vi "UI Flow Field Flow Rate.vi"(8 "error in":errorcluster) -> (0 "error out":errorcluster)   [LabVIEW 2019, in "Test.lvlib"]
uses:
  Test.lvlib
  Queues/Message Cluster.ctl
  Fluidic Process/SubVI/Fluidic Para.ctl
  LED/SubVI/Image Para.ctl
  MiControl-E/LV Source/ImageSystem/Cradle Zyla_1117/Ctl/seletion.ctl
  <vilib>/Utility/file.llb/Read Delimited Spreadsheet (string).vi
  <vilib>/Utility/error.llb/Error Cluster From Error Code.vi
  <vilib>/ErrorRing/Error Ring.xnode
  Controller/Controller.lvlib
  Queues/Queues.lvlib
  Fluidic Process/Fluidic Process.lvlib
  LED/LED.lvlib
  Motion/Allmotion/Allmotion.lvlib
  Camera/Andor/Andor.lvlib
  Image/Image.lvlib
  Initialize/Initialize.lvlib
panel:
  in  "Locate":bool
  in  "Air Tight":bool
  in  "Stop Process":bool
  out "Remaining Time(s)":dbl
  out "Total Process":string
  out "Current Process":string
  out "Gauge":dbl(knob)=1.2869315802184793e-48 scale=0.0..100.0
  in  "Purge":bool
  in  "Flow Field":bool
  in  "Flow Rate":bool
  in  "Chip Hold Pressure":bool
  in  "Back":bool
  # "/"
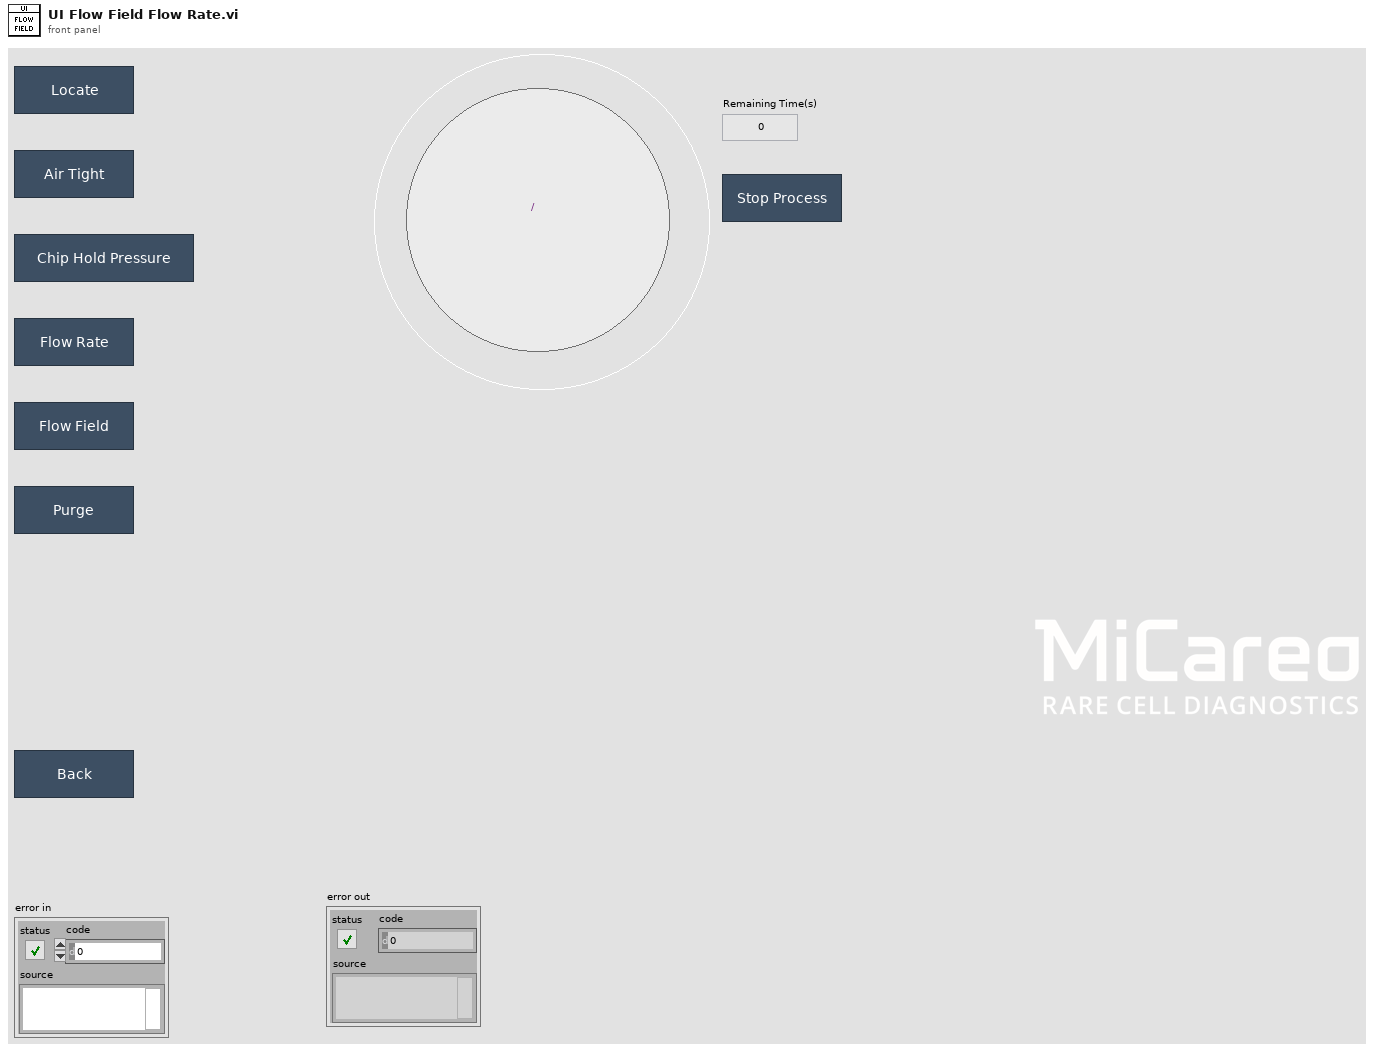
[diagram p1: front panel]
types:
  T1 = cluster{"Tick Count":u32, "Start Time":string, "Round Total":i32, "Round Count":i32, "FOV Offset":i32[], "Current Process":i32, "Take Image Done":bool}
  T2 = cluster{"Flow Field 1":refnum<queue>, "Flow Field 2":refnum<queue>}
  T3 = enum8{"Enabled", "Disabled", "Disabled and Grayed Out"}
  T4 = typedef "Fluidic Process.lvlib/Fluidic Para.ctl" = cluster{"Read Force Sensor":i32, "Read Regulator":i32, "Read Force Sensor?":bool, "Read Regulator?":bool, "Read Syringe Pump":i32, "Read Syringe Pump?":bool}
  T5 = typedef "Fluidic Process.lvlib/SEQ Data.ctl" = cluster{"Fluidic Process Done?":bool, "Current Process":i32, "Remaining Time":dbl, "Total Process":i32, "Air Sealing":bool, "Force Condition":bool}
  T6 = typedef "LED.lvlib/Image Para.ctl" = cluster{"Marker":T7, "Power(Amp)":u8, "set shutter(s)":dbl, "Cube":enum16{"1", "2", "3", "4", "5", "6", "7", "8"}}
  T7 = typedef "seletion.ctl" = enum16{"None", "Red", "Green", "Blue", "UV", "Green Laser", "Blue-Red", "UV-Red", "BF", "UV-IR"}
  T8 = typedef "ROI Descriptor" = cluster{"Global Rectangle":i32[], "Contours":cluster{"ID":enum32{"External", "Internal"}, "Type":u32, "Coordinates":i32[]}[]}
  T9 = cluster{"Image Path":path, "Start Offset":i32, "Template Path":path, "Disable Fine Search":bool, "ROI":T8}
  T10 = typedef "Rendezvous RefNum" = refnum<k1>
  T11 = typedef "Image.lvlib/SEQ Data.ctl" = cluster{"Acquire Done?":bool, "Focus Done?":bool, "Align Done?":bool, "No Position Match?":bool, "Best Wheel Position":string, "Match Done?":bool, "Match Score":dbl, "Focus Score":dbl, "Match Position":cluster{"x":sgl, "y":sgl}, "Flower Position":i32[]}
  T12 = typedef "Allmotion.lvlib/SEQ Data.ctl" = cluster{"Position":i32[], "Arrived?":bool, "VISA name":refnum<visa-resource-name>, "Initialize Done?":bool, "State":string, "VI Refnum":refnum<vi>, "Dichroic Position":string[]}
  T13 = typedef "Initialize.lvlib/SEQ Data.ctl" = cluster{"Folder Path":path}
  T14 = typedef "Andor.lvlib/SEQ Data.ctl" = cluster{"Initialize Sucess?":bool, "Image Ref":T15, "VI Refnum":refnum<vi>}
  T15 = typedef "IMAQ Image.ctl" = refnum<image>
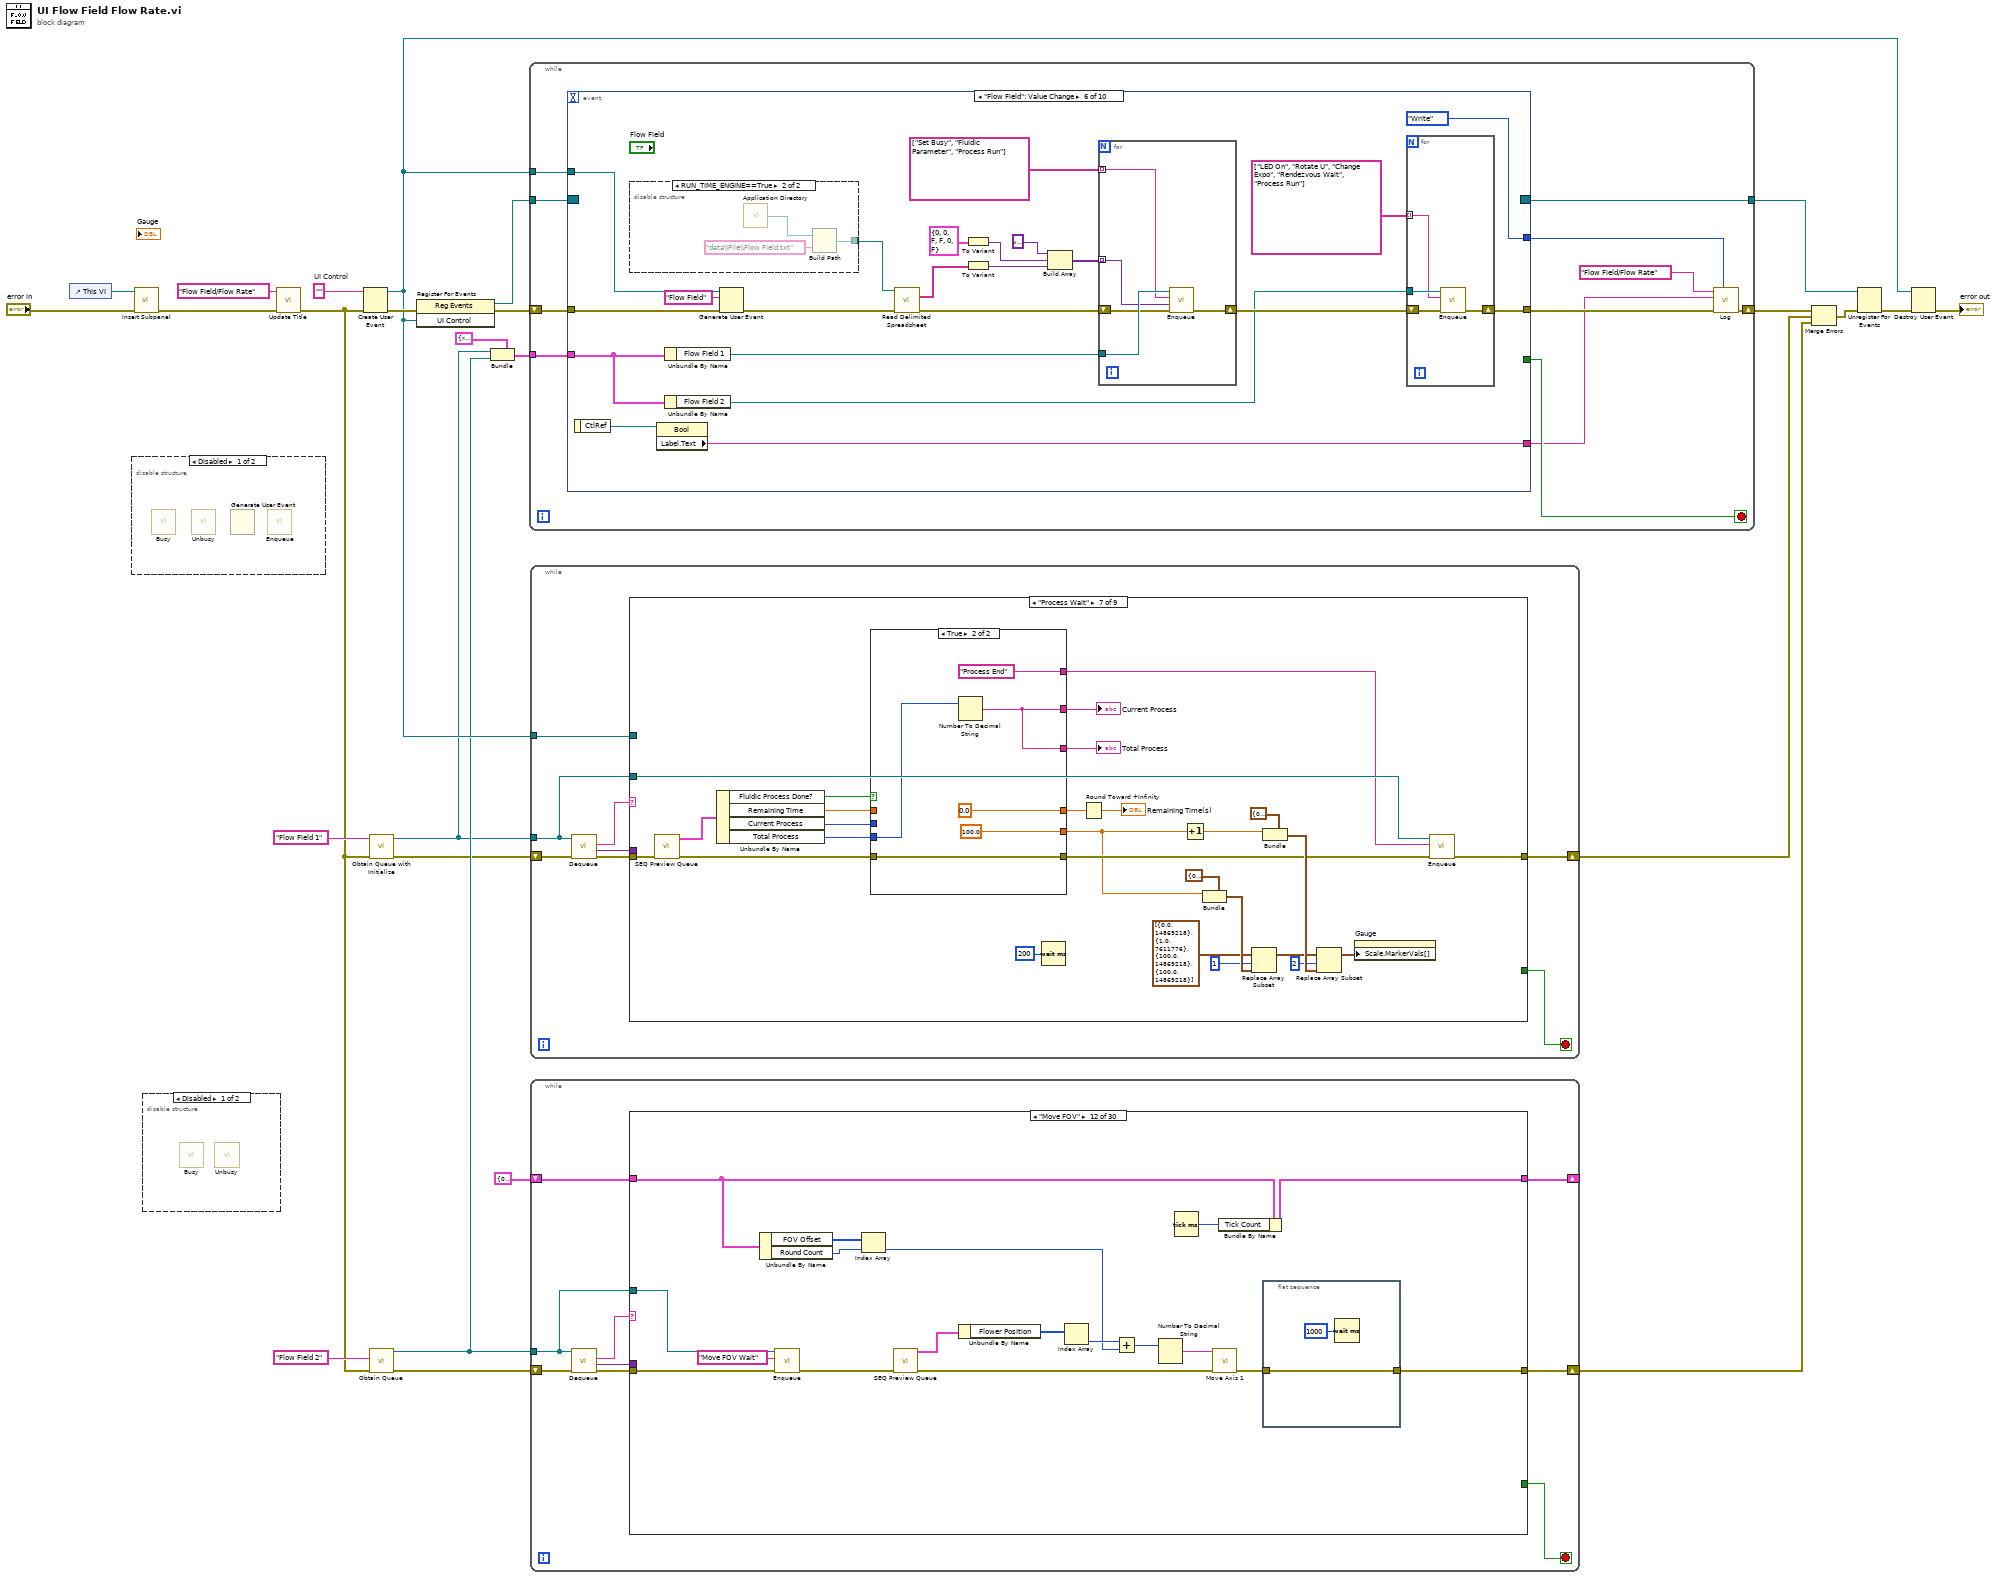
[diagram p0: block diagram]
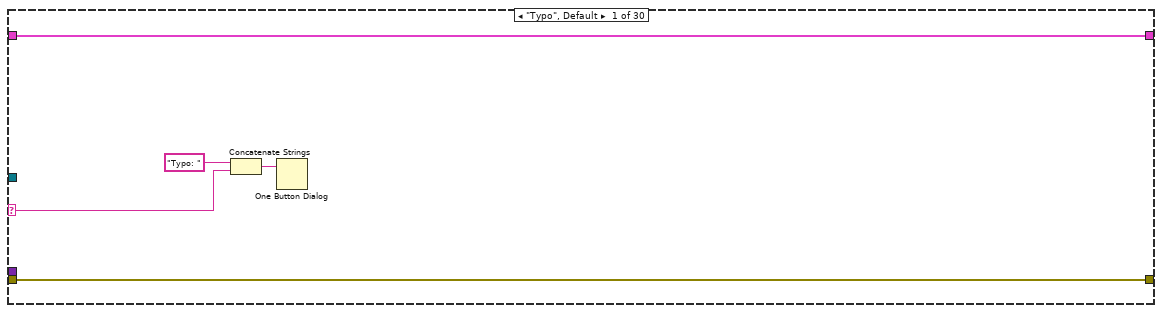
[diagram p3: hidden frame]
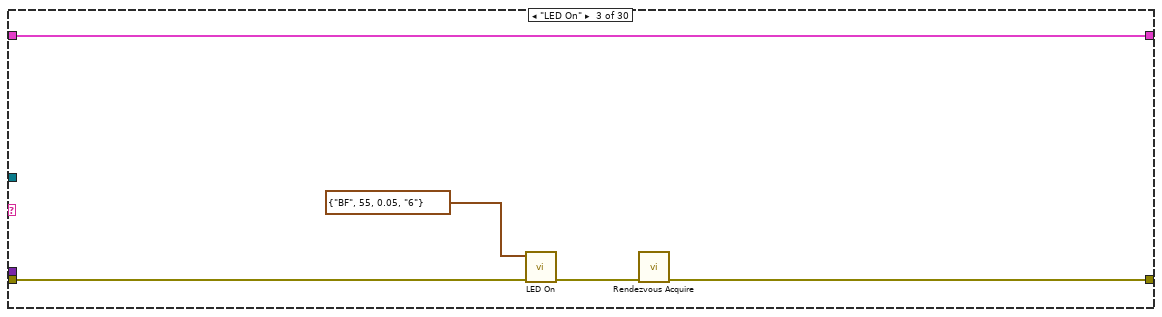
[diagram p5: hidden frame]
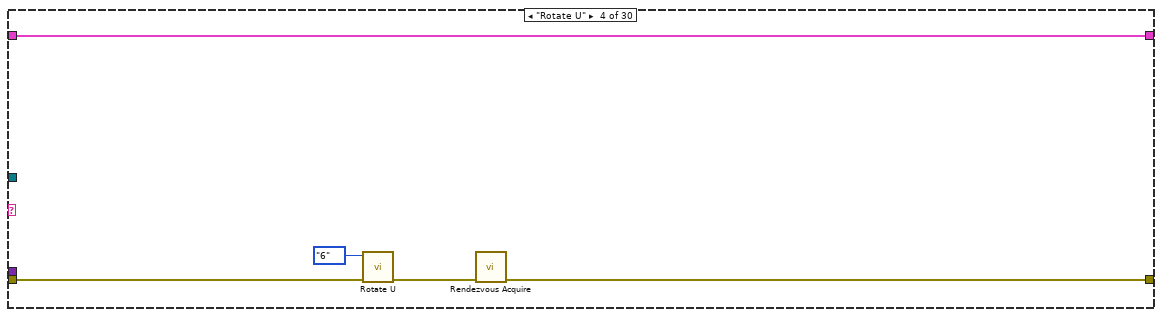
[diagram p6: hidden frame]
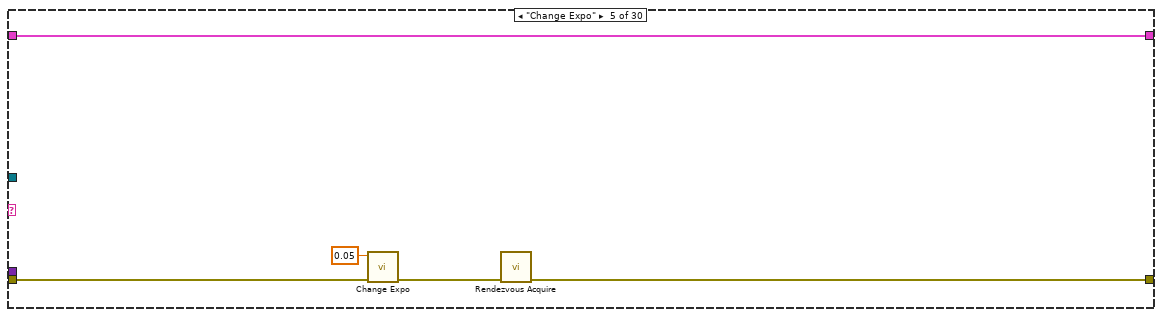
[diagram p7: hidden frame]
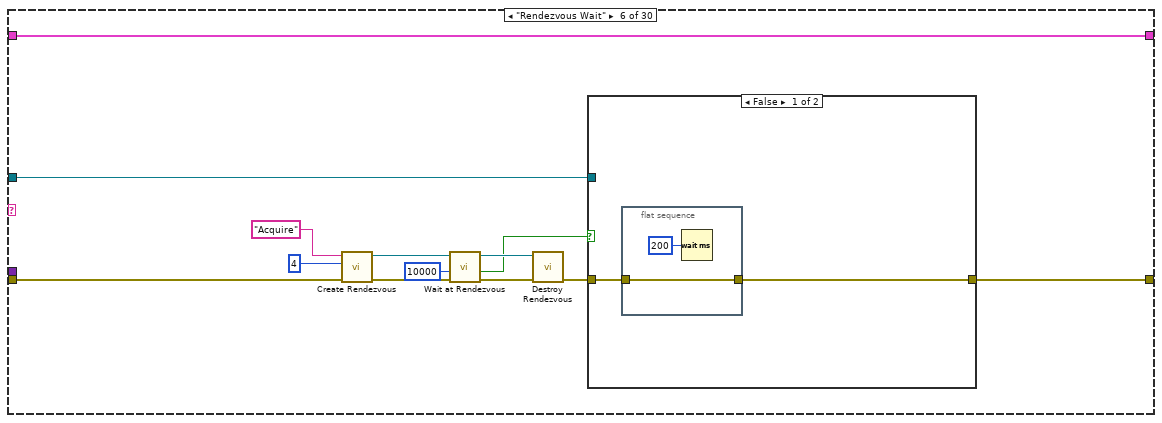
[diagram p8: hidden frame]
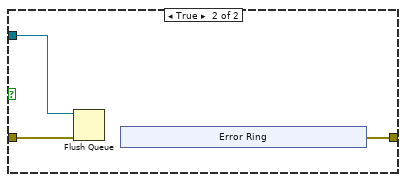
[diagram p9: hidden frame]
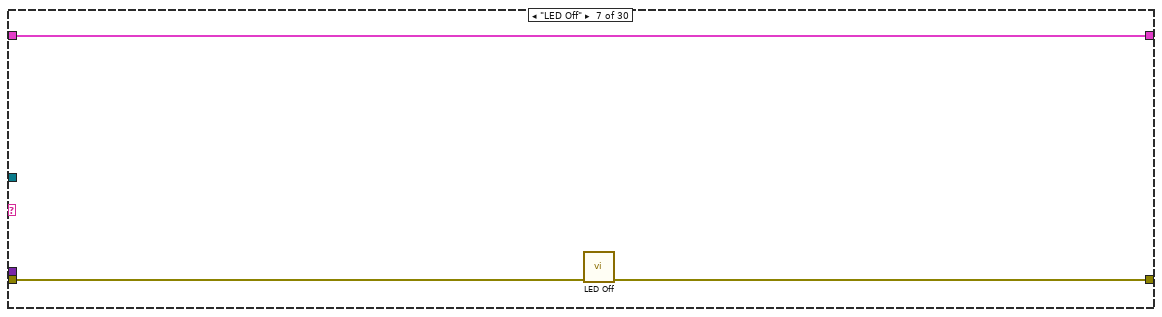
[diagram p10: hidden frame]
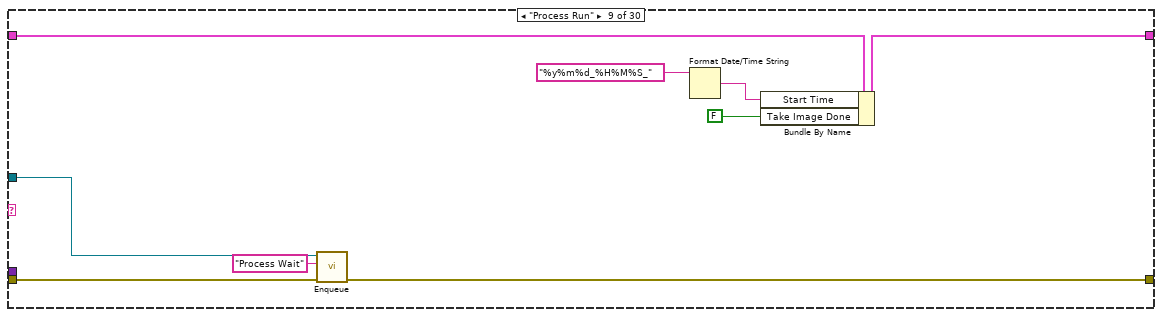
[diagram p12: hidden frame]
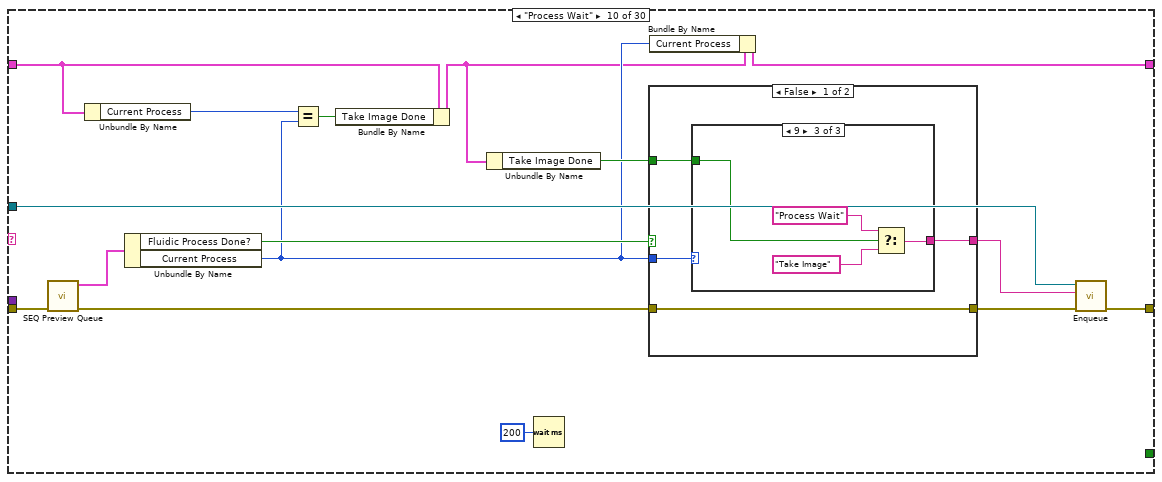
[diagram p13: hidden frame]
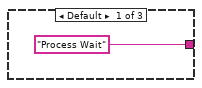
[diagram p14: hidden frame]
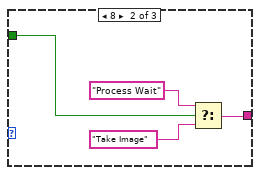
[diagram p15: hidden frame]
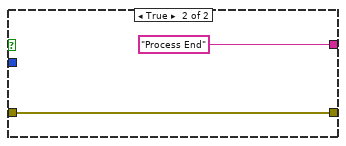
[diagram p16: hidden frame]
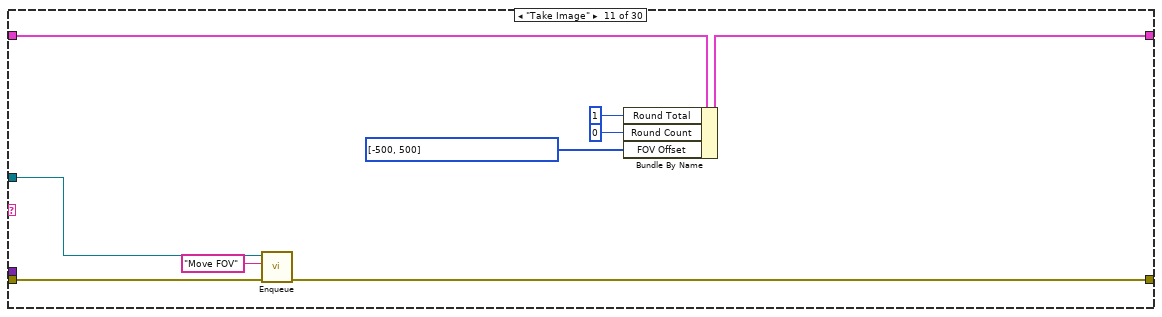
[diagram p17: hidden frame]
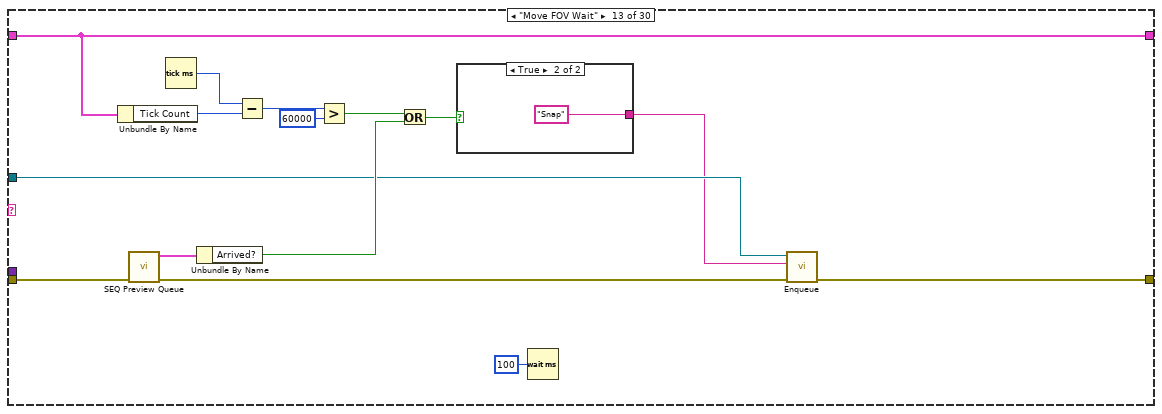
[diagram p18: hidden frame]
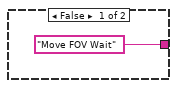
[diagram p19: hidden frame]
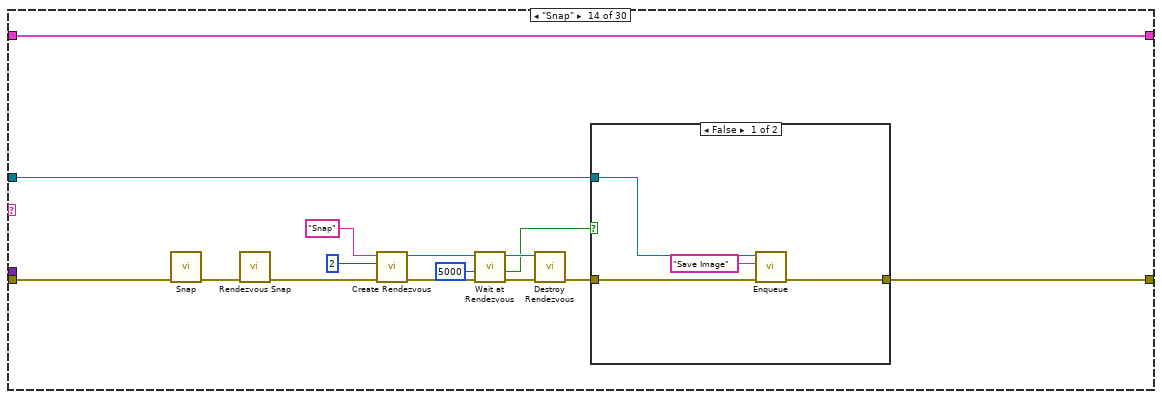
[diagram p20: hidden frame]
diagram:
  w16 = ""  # UI Control
  n1 = control-ref of="This VI"() -> (w15:refnum<vi>)
  n2 = disable-structure shown="Disabled" {
    frame Disabled {
      n3 = call "Busy.vi"() -> ()  [unwired: 11 in, 1 out]
      n4 = call "Unbusy.vi"() -> ()  [unwired: 11 in, 1 out]
      n5 = Generate User Event() -> ()  [unwired: 4 in, 2 out]
      n6 = call "Enqueue.vi"() -> ()  [unwired: 10 in, 2 out]
    }
    frame Enabled {
    }
  }
  n7 = call "Insert Subpanel.vi"("Error In"="error in", "VI Refnum"=w15) -> ("Error Out"=w3:errorcluster)  [unwired: 9 in]
  n8 = disable-structure shown="Disabled" {
    frame Disabled {
      n9 = call "Busy.vi"() -> ()  [unwired: 11 in, 1 out]
      n10 = call "Unbusy.vi"() -> ()  [unwired: 11 in, 1 out]
    }
    frame Enabled {
    }
  }
  n11 = call "Update Title.vi"("Error In"=w3, "Title"="Flow Field/Flow Rate") -> ("Error Out"=w2:errorcluster)  [unwired: 9 in]
  n12 = Create User Event(user event datatype=w16, error in=w2) -> (user event=w12:refnum<user-event>, error out=w25:errorcluster)
  n13 = call "Obtain Queue with Initialize.vi"("Error In"=w2, "Queue Name"="Flow Field 1") -> ("Error Out"=w5:errorcluster, "Queue out"=w4:refnum<queue>)  [unwired: 8 in]
  n14 = call "Obtain Queue.vi"("Error In"=w2, "Queue Name"="Flow Field 2") -> ("Error Out"=w14:errorcluster, "queue out"=w11:refnum<queue>)  [unwired: 8 in]
  n15 = register-events(error in=w25, w12) -> (reference out=w23:refnum<event-registration>, error out=w24:errorcluster)  [unwired: 1 in]
  n16 = Bundle(cluster=T2 {"Flow Field 1"=refnum, "Flow Field 2"=refnum}, "Flow Field 1"=w4, "Flow Field 2"=w11) -> (w9:T2)
  n17 = while {
    tunnel: w23 -> [w35]
    shift-right: [w30] -> w21
    shift-left: w24 -> [w37]
    tunnel: [w34] -> w19
    tunnel: w12 -> [w33]
    tunnel: w9 -> [w32]
    stop <- w36 stop-if-true
    n18 = event shown="[5] \"Flow Field\": Value Change" {
      selector: w35 -> [_ _ _ _ _ _ _ _ _ _]
      dyn-events: [_ _ _ _ _ _ _ _ _ _] -> w34
      timeout: _ -> [_ _ _ _ _ _ _ _ _ _]
      tunnel: w37 -> [w38 w43 w81 w111 w141 w175 w208 w238 w247 w253]
      tunnel: [_ w40 _ _ _ _ _ _ _ TRUE] -> w36
      tunnel: [w38 w41 w89 w119 w149 w170 w216 w237 w246 w254] -> w31
      tunnel: w33 -> [_ _ w79 w109 w139 w173 w206 _ _ _]
      tunnel: w32 -> [_ _ w77 w107 w137 w169 w204 w236 _ w252]
      tunnel: [_ _ w75 w105 w135 w165 w202 w232 w244 w249] -> w28
      tunnel: [_ enum16{"None", "Write"}."None" ("Action") enum16{"None", "Write"}."Write" ("Action") enum16{"None", "Write"}."Write" ("Action") enum16{"None", "Write"}."Write" ("Action") enum16{"None", "Write"}."Write" ("Action") enum16{"None", "Write"}."Write" ("Action") enum16{"None", "Write"}."Write" ("Action") enum16{"None", "Write"}."Write" ("Action") enum16{"None", "Write"}."Write" ("Action")] -> w27
      event Timeout {
        n19 = event-data() -> ()  [unwired: 1 in, 3 out]
      }
      event User Event {
        n20 = event-data() -> ("UI Control"=w42:string)  [unwired: 1 in]
        n21 = case shown="\"Initialize\"" w42 {
          selector: w42 -> [w46 _ _ _ _ _ _ _]
          tunnel: w43 -> [w44 w50 w54 w58 w62 w66 w70 w73]
          tunnel: [w44 w50 w54 w58 w62 w66 w70 w73] -> w41
          tunnel: [TRUE _ _ _ _ _ _ _] -> w40
          frame "Typo", Default {
            n22 = Concatenate Strings("Typo: " ("string"), w46) -> (w47:string)
            n23 = One Button Dialog(message=w47) -> ()  [unwired: 1 in, 1 out]
          }
          frame "Initialize" {
            w49 = T3."Disabled and Grayed Out" ("Disabled")
            n24 = property on="Gauge" class="Knob (strict)"("DisabledEnum"=w49) -> ()  [unwired: 2 in, 2 out]
            n25 = property on="Current Process" class="Str"("DisabledEnum"=w49) -> ()  [unwired: 2 in, 2 out]
            n26 = property on="Total Process" class="Str"("DisabledEnum"=w49) -> ()  [unwired: 2 in, 2 out]
            n27 = property on="Remaining Time(s)" class="DigNum (strict)"("DisabledEnum"=w49) -> ()  [unwired: 2 in, 2 out]
            n28 = property on="Stop Process" class="Bool"("DisabledEnum"=w49) -> ()  [unwired: 2 in, 2 out]
          }
          frame "Chip Hold Pressure" {
            w52 = T3."Enabled" ("Disabled")
            w51 = T3."Disabled and Grayed Out" ("Disabled")
            n29 = property on="Gauge" class="Knob (strict)"("DisabledEnum"=w52) -> ()  [unwired: 2 in, 2 out]
            n30 = property on="Current Process" class="Str"("DisabledEnum"=w52) -> ()  [unwired: 2 in, 2 out]
            n31 = property on="Total Process" class="Str"("DisabledEnum"=w52) -> ()  [unwired: 2 in, 2 out]
            n32 = property on="Remaining Time(s)" class="DigNum (strict)"("DisabledEnum"=w52) -> ()  [unwired: 2 in, 2 out]
            n33 = property on="Stop Process" class="Bool"("DisabledEnum"=w52) -> ()  [unwired: 2 in, 2 out]
            n34 = property on="Chip Hold Pressure" class="Bool"("DisabledEnum"=T3."Enabled" ("Disabled")) -> ()  [unwired: 2 in, 2 out]
            n35 = property on="Flow Rate" class="Bool"("DisabledEnum"=w51) -> ()  [unwired: 2 in, 2 out]
            n36 = property on="Flow Field" class="Bool"("DisabledEnum"=w51) -> ()  [unwired: 2 in, 2 out]
            n37 = property on="Purge" class="Bool"("DisabledEnum"=w51) -> ()  [unwired: 2 in, 2 out]
            n38 = property on="Air Tight" class="Bool"("DisabledEnum"=w51) -> ()  [unwired: 2 in, 2 out]
            n39 = property on="Back" class="Bool"("DisabledEnum"=w51) -> ()  [unwired: 2 in, 2 out]
            n40 = property on="Locate" class="Bool"("DisabledEnum"=w51) -> ()  [unwired: 2 in, 2 out]
          }
          frame "Air Tight" {
            w57 = T3."Enabled" ("Disabled")
            w55 = T3."Disabled and Grayed Out" ("Disabled")
            n41 = property on="Gauge" class="Knob (strict)"("DisabledEnum"=w57) -> ()  [unwired: 2 in, 2 out]
            n42 = property on="Current Process" class="Str"("DisabledEnum"=w57) -> ()  [unwired: 2 in, 2 out]
            n43 = property on="Total Process" class="Str"("DisabledEnum"=w57) -> ()  [unwired: 2 in, 2 out]
            n44 = property on="Remaining Time(s)" class="DigNum (strict)"("DisabledEnum"=w57) -> ()  [unwired: 2 in, 2 out]
            n45 = property on="Stop Process" class="Bool"("DisabledEnum"=w57) -> ()  [unwired: 2 in, 2 out]
            n46 = property on="Chip Hold Pressure" class="Bool"("DisabledEnum"=w55) -> ()  [unwired: 2 in, 2 out]
            n47 = property on="Flow Rate" class="Bool"("DisabledEnum"=w55) -> ()  [unwired: 2 in, 2 out]
            n48 = property on="Flow Field" class="Bool"("DisabledEnum"=w55) -> ()  [unwired: 2 in, 2 out]
            n49 = property on="Purge" class="Bool"("DisabledEnum"=w55) -> ()  [unwired: 2 in, 2 out]
            n50 = property on="Air Tight" class="Bool"("DisabledEnum"=T3."Enabled" ("Disabled")) -> ()  [unwired: 2 in, 2 out]
            n51 = property on="Back" class="Bool"("DisabledEnum"=w55) -> ()  [unwired: 2 in, 2 out]
            n52 = property on="Locate" class="Bool"("DisabledEnum"=w55) -> ()  [unwired: 2 in, 2 out]
          }
          frame "Flow Rate" {
            w60 = T3."Enabled" ("Disabled")
            w59 = T3."Disabled and Grayed Out" ("Disabled")
            n53 = property on="Gauge" class="Knob (strict)"("DisabledEnum"=w60) -> ()  [unwired: 2 in, 2 out]
            n54 = property on="Current Process" class="Str"("DisabledEnum"=w60) -> ()  [unwired: 2 in, 2 out]
            n55 = property on="Total Process" class="Str"("DisabledEnum"=w60) -> ()  [unwired: 2 in, 2 out]
            n56 = property on="Remaining Time(s)" class="DigNum (strict)"("DisabledEnum"=w60) -> ()  [unwired: 2 in, 2 out]
            n57 = property on="Stop Process" class="Bool"("DisabledEnum"=w60) -> ()  [unwired: 2 in, 2 out]
            n58 = property on="Chip Hold Pressure" class="Bool"("DisabledEnum"=w59) -> ()  [unwired: 2 in, 2 out]
            n59 = property on="Flow Rate" class="Bool"("DisabledEnum"=T3."Enabled" ("Disabled")) -> ()  [unwired: 2 in, 2 out]
            n60 = property on="Flow Field" class="Bool"("DisabledEnum"=w59) -> ()  [unwired: 2 in, 2 out]
            n61 = property on="Purge" class="Bool"("DisabledEnum"=w59) -> ()  [unwired: 2 in, 2 out]
            n62 = property on="Air Tight" class="Bool"("DisabledEnum"=w59) -> ()  [unwired: 2 in, 2 out]
            n63 = property on="Back" class="Bool"("DisabledEnum"=w59) -> ()  [unwired: 2 in, 2 out]
            n64 = property on="Locate" class="Bool"("DisabledEnum"=w59) -> ()  [unwired: 2 in, 2 out]
          }
          frame "Flow Field" {
            w64 = T3."Enabled" ("Disabled")
            w63 = T3."Disabled and Grayed Out" ("Disabled")
            n65 = property on="Gauge" class="Knob (strict)"("DisabledEnum"=w64) -> ()  [unwired: 2 in, 2 out]
            n66 = property on="Current Process" class="Str"("DisabledEnum"=w64) -> ()  [unwired: 2 in, 2 out]
            n67 = property on="Total Process" class="Str"("DisabledEnum"=w64) -> ()  [unwired: 2 in, 2 out]
            n68 = property on="Remaining Time(s)" class="DigNum (strict)"("DisabledEnum"=w64) -> ()  [unwired: 2 in, 2 out]
            n69 = property on="Stop Process" class="Bool"("DisabledEnum"=w64) -> ()  [unwired: 2 in, 2 out]
            n70 = property on="Chip Hold Pressure" class="Bool"("DisabledEnum"=w63) -> ()  [unwired: 2 in, 2 out]
            n71 = property on="Flow Rate" class="Bool"("DisabledEnum"=w63) -> ()  [unwired: 2 in, 2 out]
            n72 = property on="Flow Field" class="Bool"("DisabledEnum"=T3."Enabled" ("Disabled")) -> ()  [unwired: 2 in, 2 out]
            n73 = property on="Purge" class="Bool"("DisabledEnum"=w63) -> ()  [unwired: 2 in, 2 out]
            n74 = property on="Air Tight" class="Bool"("DisabledEnum"=w63) -> ()  [unwired: 2 in, 2 out]
            n75 = property on="Back" class="Bool"("DisabledEnum"=w63) -> ()  [unwired: 2 in, 2 out]
            n76 = property on="Locate" class="Bool"("DisabledEnum"=w63) -> ()  [unwired: 2 in, 2 out]
          }
          frame "Purge" {
            w68 = T3."Enabled" ("Disabled")
            w67 = T3."Disabled and Grayed Out" ("Disabled")
            n77 = property on="Gauge" class="Knob (strict)"("DisabledEnum"=w68) -> ()  [unwired: 2 in, 2 out]
            n78 = property on="Current Process" class="Str"("DisabledEnum"=w68) -> ()  [unwired: 2 in, 2 out]
            n79 = property on="Total Process" class="Str"("DisabledEnum"=w68) -> ()  [unwired: 2 in, 2 out]
            n80 = property on="Remaining Time(s)" class="DigNum (strict)"("DisabledEnum"=w68) -> ()  [unwired: 2 in, 2 out]
            n81 = property on="Stop Process" class="Bool"("DisabledEnum"=w68) -> ()  [unwired: 2 in, 2 out]
            n82 = property on="Chip Hold Pressure" class="Bool"("DisabledEnum"=w67) -> ()  [unwired: 2 in, 2 out]
            n83 = property on="Flow Rate" class="Bool"("DisabledEnum"=w67) -> ()  [unwired: 2 in, 2 out]
            n84 = property on="Flow Field" class="Bool"("DisabledEnum"=w67) -> ()  [unwired: 2 in, 2 out]
            n85 = property on="Purge" class="Bool"("DisabledEnum"=T3."Enabled" ("Disabled")) -> ()  [unwired: 2 in, 2 out]
            n86 = property on="Air Tight" class="Bool"("DisabledEnum"=w67) -> ()  [unwired: 2 in, 2 out]
            n87 = property on="Back" class="Bool"("DisabledEnum"=w67) -> ()  [unwired: 2 in, 2 out]
            n88 = property on="Locate" class="Bool"("DisabledEnum"=w67) -> ()  [unwired: 2 in, 2 out]
          }
          frame "Process End" {
            w72 = T3."Disabled and Grayed Out" ("Disabled")
            w71 = T3."Enabled" ("Disabled")
            n89 = property on="Gauge" class="Knob (strict)"("DisabledEnum"=w72) -> ()  [unwired: 2 in, 2 out]
            n90 = property on="Current Process" class="Str"("DisabledEnum"=w72) -> ()  [unwired: 2 in, 2 out]
            n91 = property on="Total Process" class="Str"("DisabledEnum"=w72) -> ()  [unwired: 2 in, 2 out]
            n92 = property on="Remaining Time(s)" class="DigNum (strict)"("DisabledEnum"=w72) -> ()  [unwired: 2 in, 2 out]
            n93 = property on="Stop Process" class="Bool"("DisabledEnum"=w72) -> ()  [unwired: 2 in, 2 out]
            n94 = property on="Chip Hold Pressure" class="Bool"("DisabledEnum"=w71) -> ()  [unwired: 2 in, 2 out]
            n95 = property on="Flow Rate" class="Bool"("DisabledEnum"=w71) -> ()  [unwired: 2 in, 2 out]
            n96 = property on="Flow Field" class="Bool"("DisabledEnum"=w71) -> ()  [unwired: 2 in, 2 out]
            n97 = property on="Purge" class="Bool"("DisabledEnum"=w71) -> ()  [unwired: 2 in, 2 out]
            n98 = property on="Air Tight" class="Bool"("DisabledEnum"=w71) -> ()  [unwired: 2 in, 2 out]
            n99 = property on="Back" class="Bool"("DisabledEnum"=w71) -> ()  [unwired: 2 in, 2 out]
            n100 = property on="Locate" class="Bool"("DisabledEnum"=w71) -> ()  [unwired: 2 in, 2 out]
          }
        }
      }
      event "Chip Hold Pressure": Value Change {
        n101 = event-data() -> ("CtlRef"=w76:refnum<vi>)  [unwired: 1 in]
        n102 = property class="Bool"(reference=w76) -> ("Label.Text"=w75:string)  [unwired: 1 in, 2 out]
        n103 = Unbundle By Name(w77) -> ("Flow Field 1"=w78:refnum<queue>)
        n104 = disable-structure shown="RUN_TIME_ENGINE==True" {
          disable-tunnel: [w93 w96] -> w91
          frame condition #0 (active) {
            n105 = call <vilib>:"Application Directory.vi"() -> ("Application Directory"=w95:path)
            n106 = Build Path(base path=w95, name or relative path="Fluidic Process\\File\\Chip Hold Pressure.txt") -> (appended path=w93:path)
          }
          frame condition #1 {
            n107 = call <vilib>:"Application Directory.vi"() -> ("Application Directory"=w98:path)
            n108 = Build Path(base path=w98, name or relative path="data\\File\\Chip Hold Pressure.txt") -> (appended path=w96:path)
          }
        }
        n109 = Generate User Event(user event=w79, event data cluster="Chip Hold Pressure" ("event data"), error in=w81) -> (error out=w80:errorcluster)  [unwired: 1 in, 1 out]
        n110 = call-poly <vilib>:"Read Delimited Spreadsheet.vi"("file path (dialog if empty)"=w91, "error in (no error)"=w80) -> ("all rows"=w90:string[][], "error out"=w92:errorcluster)  [unwired: 8 in, 4 out]
        n111 = To Variant(anything=T4 {"Read Force Sensor"=0, "Read Regulator"=0, "Read Force Sensor?"=FALSE, "Read Regulator?"=FALSE, "Read Syringe Pump"=0, "Read Syringe Pump?"=FALSE} ("Cluster")) -> (Variant=w85:variant)
        n112 = To Variant(anything=w90) -> (Variant=w87:variant)
        n113 = Build Array(variant, w85, w87) -> (w84:variant[])
        n114 = for {
          tunnel: w78 -> [w103]
          shift-right: [w101] -> w89
          shift-left: w92 -> [w102]
          tunnel: string[] ["Set Busy", "Fluidic Parameter", "Process Run"] -> [w100] mode=indexing
          tunnel: w84 -> [w99] mode=indexing
          n115 = call "Enqueue.vi"("Error In"=w102, "Data"=w99, "State"=w100, "Queue in"=w103) -> ("Error Out"=w101:errorcluster)  [unwired: 6 in, 1 out]
        }
      }
      event "Air Tight": Value Change {
        n116 = event-data() -> ("CtlRef"=w106:refnum<vi>)  [unwired: 1 in]
        n117 = Unbundle By Name(w107) -> ("Flow Field 1"=w108:refnum<queue>)
        n118 = property class="Bool"(reference=w106) -> ("Label.Text"=w105:string)  [unwired: 1 in, 2 out]
        n119 = Generate User Event(user event=w109, event data cluster="Air Tight" ("event data"), error in=w111) -> (error out=w110:errorcluster)  [unwired: 1 in, 1 out]
        n120 = disable-structure shown="RUN_TIME_ENGINE==False, Default" {
          disable-tunnel: [w123 w126] -> w121
          frame condition #0 (active) {
            n121 = call <vilib>:"Application Directory.vi"() -> ("Application Directory"=w125:path)
            n122 = Build Path(base path=w125, name or relative path="Fluidic Process\\File\\Air Tight.txt") -> (appended path=w123:path)
          }
          frame condition #1 {
            n123 = call <vilib>:"Application Directory.vi"() -> ("Application Directory"=w128:path)
            n124 = Build Path(base path=w128, name or relative path="data\\File\\Air Tight.txt") -> (appended path=w126:path)
          }
        }
        n125 = call-poly <vilib>:"Read Delimited Spreadsheet.vi"("file path (dialog if empty)"=w121, "error in (no error)"=w110) -> ("all rows"=w120:string[][], "error out"=w122:errorcluster)  [unwired: 8 in, 4 out]
        n126 = To Variant(anything=T4 {"Read Force Sensor"=0, "Read Regulator"=2, "Read Force Sensor?"=FALSE, "Read Regulator?"=TRUE, "Read Syringe Pump"=0, "Read Syringe Pump?"=FALSE} ("Cluster")) -> (Variant=w115:variant)
        n127 = To Variant(anything=w120) -> (Variant=w117:variant)
        n128 = Build Array(variant, w115, w117) -> (w114:variant[])
        n129 = for {
          tunnel: w108 -> [w133]
          shift-right: [w131] -> w119
          shift-left: w122 -> [w132]
          tunnel: string[] ["Set Busy", "Fluidic Parameter", "Process Run"] -> [w130] mode=indexing
          tunnel: w114 -> [w129] mode=indexing
          n130 = call "Enqueue.vi"("Error In"=w132, "Data"=w129, "State"=w130, "Queue in"=w133) -> ("Error Out"=w131:errorcluster)  [unwired: 6 in, 1 out]
        }
      }
      event "Flow Rate": Value Change {
        n131 = event-data() -> ("CtlRef"=w136:refnum<vi>)  [unwired: 1 in]
        n132 = Unbundle By Name(w137) -> ("Flow Field 1"=w138:refnum<queue>)
        n133 = property class="Bool"(reference=w136) -> ("Label.Text"=w135:string)  [unwired: 1 in, 2 out]
        n134 = Generate User Event(user event=w139, event data cluster="Flow Rate" ("event data"), error in=w141) -> (error out=w140:errorcluster)  [unwired: 1 in, 1 out]
        n135 = disable-structure shown="RUN_TIME_ENGINE==True" {
          disable-tunnel: [w153 w156] -> w151
          frame condition #0 (active) {
            n136 = call <vilib>:"Application Directory.vi"() -> ("Application Directory"=w155:path)
            n137 = Build Path(base path=w155, name or relative path="Fluidic Process\\File\\Flow Rate.txt") -> (appended path=w153:path)
          }
          frame condition #1 {
            n138 = call <vilib>:"Application Directory.vi"() -> ("Application Directory"=w158:path)
            n139 = Build Path(base path=w158, name or relative path="data\\File\\Flow Rate.txt") -> (appended path=w156:path)
          }
        }
        n140 = call-poly <vilib>:"Read Delimited Spreadsheet.vi"("file path (dialog if empty)"=w151, "error in (no error)"=w140) -> ("all rows"=w150:string[][], "error out"=w152:errorcluster)  [unwired: 8 in, 4 out]
        n141 = To Variant(anything=T4 {"Read Force Sensor"=0, "Read Regulator"=0, "Read Force Sensor?"=FALSE, "Read Regulator?"=FALSE, "Read Syringe Pump"=0, "Read Syringe Pump?"=FALSE} ("Cluster")) -> (Variant=w145:variant)
        n142 = To Variant(anything=w150) -> (Variant=w147:variant)
        n143 = Build Array(variant, w145, w147) -> (w144:variant[])
        n144 = for {
          tunnel: w138 -> [w163]
          shift-right: [w161] -> w149
          shift-left: w152 -> [w162]
          tunnel: string[] ["Set Busy", "Fluidic Parameter", "Process Run"] -> [w160] mode=indexing
          tunnel: w144 -> [w159] mode=indexing
          n145 = call "Enqueue.vi"("Error In"=w162, "Data"=w159, "State"=w160, "Queue in"=w163) -> ("Error Out"=w161:errorcluster)  [unwired: 6 in, 1 out]
        }
      }
      event "Flow Field": Value Change {
        n146 = event-data() -> ("CtlRef"=w166:refnum<vi>)  [unwired: 1 in]
        n147 = disable-structure shown="RUN_TIME_ENGINE==True" {
          disable-tunnel: [w190 w193] -> w184
          frame condition #0 (active) {
            n148 = call <vilib>:"Application Directory.vi"() -> ("Application Directory"=w192:path)
            n149 = Build Path(base path=w192, name or relative path="Fluidic Process\\File\\Flow Field.txt") -> (appended path=w190:path)
          }
          frame condition #1 {
            n150 = call <vilib>:"Application Directory.vi"() -> ("Application Directory"=w195:path)
            n151 = Build Path(base path=w195, name or relative path="data\\File\\Flow Field.txt") -> (appended path=w193:path)
          }
        }
        n152 = property class="Bool"(reference=w166) -> ("Label.Text"=w165:string)  [unwired: 1 in, 2 out]
        n153 = Unbundle By Name(w169) -> ("Flow Field 1"=w172:refnum<queue>)
        n154 = Unbundle By Name(w169) -> ("Flow Field 2"=w168:refnum<queue>)
        n155 = Generate User Event(user event=w173, event data cluster="Flow Field" ("event data"), error in=w175) -> (error out=w174:errorcluster)  [unwired: 1 in, 1 out]
        n156 = call-poly <vilib>:"Read Delimited Spreadsheet.vi"("file path (dialog if empty)"=w184, "error in (no error)"=w174) -> ("all rows"=w183:string[][], "error out"=w185:errorcluster)  [unwired: 8 in, 4 out]
        n157 = To Variant(anything=T4 {"Read Force Sensor"=0, "Read Regulator"=0, "Read Force Sensor?"=FALSE, "Read Regulator?"=FALSE, "Read Syringe Pump"=0, "Read Syringe Pump?"=FALSE} ("Cluster")) -> (Variant=w179:variant)
        n158 = To Variant(anything=w183) -> (Variant=w181:variant)
        n159 = Build Array(variant, w179, w181) -> (w178:variant[])
        n160 = for {
          tunnel: w172 -> [w200]
          shift-right: [w198] -> w171
          shift-left: w185 -> [w199]
          tunnel: string[] ["Set Busy", "Fluidic Parameter", "Process Run"] -> [w197] mode=indexing
          tunnel: w178 -> [w196] mode=indexing
          n161 = call "Enqueue.vi"("Error In"=w199, "Data"=w196, "State"=w197, "Queue in"=w200) -> ("Error Out"=w198:errorcluster)  [unwired: 6 in, 1 out]
        }
        n162 = for {
          tunnel: w168 -> [w187]
          shift-right: [w188] -> w170
          shift-left: w171 -> [w189]
          tunnel: string[] ["LED On", "Rotate U", "Change Expo", "Rendezvous Wait", "Process Run"] -> [w186] mode=indexing
          n163 = call "Enqueue.vi"("Error In"=w189, "State"=w186, "Queue in"=w187) -> ("Error Out"=w188:errorcluster)  [unwired: 7 in, 1 out]
        }
      }
      event "Purge": Value Change {
        n164 = event-data() -> ("CtlRef"=w203:refnum<vi>)  [unwired: 1 in]
        n165 = property class="Bool"(reference=w203) -> ("Label.Text"=w202:string)  [unwired: 1 in, 2 out]
        n166 = Unbundle By Name(w204) -> ("Flow Field 1"=w205:refnum<queue>)
        n167 = Generate User Event(user event=w206, event data cluster="Purge" ("event data"), error in=w208) -> (error out=w207:errorcluster)  [unwired: 1 in, 1 out]
        n168 = disable-structure shown="RUN_TIME_ENGINE==False, Default" {
          disable-tunnel: [w220 w223] -> w218
          frame condition #0 (active) {
            n169 = call <vilib>:"Application Directory.vi"() -> ("Application Directory"=w222:path)
            n170 = Build Path(base path=w222, name or relative path="Fluidic Process\\File\\Purge.txt") -> (appended path=w220:path)
          }
          frame condition #1 {
            n171 = call <vilib>:"Application Directory.vi"() -> ("Application Directory"=w225:path)
            n172 = Build Path(base path=w225, name or relative path="data\\File\\Purge.txt") -> (appended path=w223:path)
          }
        }
        n173 = call-poly <vilib>:"Read Delimited Spreadsheet.vi"("file path (dialog if empty)"=w218, "error in (no error)"=w207) -> ("all rows"=w217:string[][], "error out"=w219:errorcluster)  [unwired: 8 in, 4 out]
        n174 = To Variant(anything=T4 {"Read Force Sensor"=0, "Read Regulator"=0, "Read Force Sensor?"=FALSE, "Read Regulator?"=FALSE, "Read Syringe Pump"=3, "Read Syringe Pump?"=TRUE} ("Cluster")) -> (Variant=w212:variant)
        n175 = To Variant(anything=w217) -> (Variant=w214:variant)
        n176 = Build Array(variant, w212, w214) -> (w211:variant[])
        n177 = for {
          tunnel: w205 -> [w230]
          shift-right: [w228] -> w216
          shift-left: w219 -> [w229]
          tunnel: string[] ["Set Busy", "Fluidic Parameter", "Process Run"] -> [w227] mode=indexing
          tunnel: w211 -> [w226] mode=indexing
          n178 = call "Enqueue.vi"("Error In"=w229, "Data"=w226, "State"=w227, "Queue in"=w230) -> ("Error Out"=w228:errorcluster)  [unwired: 6 in, 1 out]
        }
      }
      event "Locate": Value Change {
        n179 = event-data() -> ("CtlRef"=w233:refnum<vi>)  [unwired: 1 in]
        n180 = property class="Bool"(reference=w233) -> ("Label.Text"=w232:string)  [unwired: 1 in, 2 out]
        n181 = Unbundle By Name(w236) -> ("Flow Field 2"=w235:refnum<queue>)
        n182 = for {
          tunnel: w235 -> [w240]
          shift-right: [w241] -> w237
          shift-left: w238 -> [w242]
          tunnel: string[] ["LED On", "Rotate U", "Change Expo", "Rendezvous Wait", "Go Reference"] -> [w239] mode=indexing
          n183 = call "Enqueue.vi"("Error In"=w242, "State"=w239, "Queue in"=w240) -> ("Error Out"=w241:errorcluster)  [unwired: 7 in, 1 out]
        }
      }
      event "Stop Process": Value Change {
        n184 = event-data() -> ("CtlRef"=w245:refnum<vi>)  [unwired: 1 in]
        n185 = property class="Bool"(reference=w245) -> ("Label.Text"=w244:string)  [unwired: 1 in, 2 out]
        n186 = call "Stop Process.vi"("Error In"=w247) -> ("Error Out"=w246:errorcluster)  [unwired: 10 in]
      }
      event "Back": Value Change {
        n187 = event-data() -> ("CtlRef"=w250:refnum<vi>)  [unwired: 1 in]
        n188 = property class="Bool"(reference=w250) -> ("Label.Text"=w249:string)  [unwired: 1 in, 2 out]
        n189 = Cluster To Array(cluster=w252) -> (array=w251:refnum<queue>[])
        n190 = for {
          shift-right: [w259] -> w254
          shift-left: w253 -> [w258]
          tunnel: w251 -> [w257] mode=indexing
          n191 = call "Enqueue.vi"("Error In"=w258, "State"="Close", "Queue in"=w257) -> ("Error Out"=w259:errorcluster)  [unwired: 7 in, 1 out]
        }
      }
    }
    n192 = call "Log.vi"("Action"=w27, "error in"=w31, "State"=w28, "Page Name"="Flow Field/Flow Rate") -> ("error out"=w30:errorcluster)  [unwired: 7 in]
  }
  n193 = while {
    tunnel: w4 -> [w264]
    shift-right: [w262] -> w20
    shift-left: w5 -> [w267]
    tunnel: w12 -> [w261]
    stop <- w260 stop-if-true
    n194 = call "Dequeue.vi"("Error In"=w267, "Queue in"=w264) -> ("Error Out"=w263:errorcluster, "Data"=w265:variant, "State"=w266:string)  [unwired: 6 in, 1 out]
    n195 = case shown="\"Process Wait\"" w266 {
      selector: w266 -> [w269 _ _ _ _ _ _ _ _]
      tunnel: w265 -> [_ _ _ w282 w292 _ _ _ _]
      tunnel: w264 -> [_ _ _ _ w287 w299 w306 _ w349]
      tunnel: w263 -> [w268 w275 w277 w283 w293 w300 w327 w347 w351]
      tunnel: [_ _ _ _ _ _ _ _ TRUE] -> w260
      tunnel: [w268 w274 w276 w278 w284 w296 w311 w346 w350] -> w262
      tunnel: w261 -> [_ w273 _ _ _ _ _ w345 _]
      frame "Typo", Default {
        n196 = Concatenate Strings("Typo: " ("string"), w269) -> (w271:string)
        n197 = One Button Dialog(message=w271) -> ()  [unwired: 1 in, 1 out]
      }
      frame "Initialize" {
        n198 = Generate User Event(user event=w273, event data cluster="Initialize" ("event data"), error in=w275) -> (error out=w274:errorcluster)  [unwired: 1 in, 1 out]
      }
      frame "Set Busy" {
        n199 = call "Busy.vi"("Error In"=w277) -> ("Error Out"=w276:errorcluster)  [unwired: 10 in]
      }
      frame "Fluidic Parameter" {
        n200 = Variant To Data(error in=w283, type=T4 {"Read Force Sensor"=0, "Read Regulator"=0, "Read Force Sensor?"=FALSE, "Read Regulator?"=FALSE, "Read Syringe Pump"=0, "Read Syringe Pump?"=FALSE} ("Cluster"), Variant=w282) -> (data=w279:T4, error out=w280:errorcluster)
        n201 = call "Update Fluidic Para.vi"("Error In"=w280, "Fluidic Para"=w279) -> ("Error Out"=w278:errorcluster)  [unwired: 9 in]
      }
      frame "Process Run" {
        n202 = Variant To Data(error in=w293, type=string[][] [] ("all rows"), Variant=w292) -> (data=w289:string[][], error out=w290:errorcluster)
        n203 = call "Run Process.vi"("Error In"=w290, "Fluidic Process in"=w289) -> ("Error Out"=w288:errorcluster)  [unwired: 9 in]
        n204 = call "Enqueue.vi"("Error In"=w288, "State"="Unset Busy", "Queue in"=w287) -> ("Error Out"=w285:errorcluster)  [unwired: 7 in, 1 out]
        n205 = flat-sequence {
          tunnel: w285 -> [w295]
          tunnel: [w295] -> w284
          frame #0 {
            n206 = Wait (ms)(milliseconds to wait=u32 1000) -> ()  [unwired: 1 out]
          }
        }
      }
      frame "Unset Busy" {
        n207 = call "Enqueue.vi"("Error In"=w300, "State"="Process Wait", "Queue in"=w299) -> ("Error Out"=w297:errorcluster)  [unwired: 7 in, 1 out]
        n208 = call "Unbusy.vi"("Error In"=w297) -> ("Error Out"=w296:errorcluster)  [unwired: 10 in]
      }
      frame "Process Wait" {
        n209 = call "SEQ Preview Queue.vi"("error in"=w327) -> ("error out"=w324:errorcluster, "SEQ Data"=w326:T5)  [unwired: 9 in]
        n210 = Unbundle By Name(w326) -> ("Fluidic Process Done?"=w325:bool, "Remaining Time"=w310:dbl, "Current Process"=w309:i32, "Total Process"=w308:i32)
        n211 = case shown="True" w325 {
          tunnel: w324 -> [w335 w343]
          tunnel: [w335 w343] -> w312
          tunnel: w310 -> [w334 _]
          tunnel: w309 -> [w332 _]
          tunnel: w308 -> [w331 w342]
          tunnel: [w334 0.0 ("Remaining Time")] -> w302
          tunnel: [w333 100.0] -> w307
          tunnel: [w330 w341] -> w305
          tunnel: [w329 w341] -> w304
          tunnel: ["Process Wait" "Process End"] -> w303
          frame False {
            n212 = Divide(x=w332, y=w331) -> (x/y=w337:dbl)
            n213 = Number To Decimal String(number=w332) -> (decimal integer string=w330:string)  [unwired: 1 in]
            n214 = Number To Decimal String(number=w331) -> (decimal integer string=w329:string)  [unwired: 1 in]
            n215 = Multiply(x=w337, y=100.0) -> (x*y=w333:dbl)
          }
          frame True {
            n216 = Number To Decimal String(number=w342) -> (decimal integer string=w341:string)  [unwired: 1 in]
          }
        }
        "Total Process" <- w304
        "Current Process" <- w305
        n217 = Wait (ms)(milliseconds to wait=u32 200) -> ()  [unwired: 1 out]
        n218 = Round Toward +Infinity(x=w302) -> (ceil(x): smallest int >= x=→"Remaining Time(s)":dbl)
        n219 = Increment(x=w307) -> (x+1=w320:dbl)
        n220 = Bundle(cluster=cluster{dbl, i32} {0.0, 7611776}, w307) -> (w319:cluster{dbl, i32})  [unwired: 1 in]
        n221 = Replace Array Subset(array=cluster{dbl, u32}[] [{0.0, 14869218}, {1.0, 7611776}, {100.0, 14869218}, {100.0, 14869218}] ("Scale.Marker Values[]"), new element=w319, index=1) -> (w321:cluster{dbl, u32}[])
        n222 = Bundle(cluster=cluster{dbl, i32} {0.0, 14869218}, w320) -> (w322:cluster{dbl, i32})  [unwired: 1 in]
        n223 = Replace Array Subset(array=w321, new element=w322, index=2) -> (w323:cluster{dbl, u32}[])
        n224 = property on="Gauge" class="Knob (strict)"("Scale.MarkerVals[]"=w323) -> ()  [unwired: 2 in, 2 out]
        n225 = call "Enqueue.vi"("Error In"=w312, "State"=w303, "Queue in"=w306) -> ("Error Out"=w311:errorcluster)  [unwired: 7 in, 1 out]
      }
      frame "Process End" {
        n226 = Generate User Event(user event=w345, event data cluster="Process End" ("event data"), error in=w347) -> (error out=w346:errorcluster)  [unwired: 1 in, 1 out]
        n227 = call "Process Msg"() -> ()  [unwired: 10 in, 2 out]
      }
      frame "Close" {
        n228 = Release Queue(queue=w349, error in (no error)=w351) -> (error out=w350:errorcluster)  [unwired: 1 in, 2 out]
      }
    }
  }
  n229 = while {
    tunnel: w11 -> [w357]
    shift-right: [w355] -> w7
    shift-left: w14 -> [w360]
    shift-right: [w352] -> _
    shift-left: T1 {"Tick Count"=0, "Start Time"="", "Round Total"=0, "Round Count"=0, "FOV Offset"=[], "Current Process"=0, "Take Image Done"=FALSE} -> [w353]
    stop <- w354 stop-if-true
    n230 = call "Dequeue.vi"("Error In"=w360, "Queue in"=w357) -> ("Error Out"=w356:errorcluster, "Data"=w358:variant, "State"=w359:string)  [unwired: 6 in, 1 out]
    n231 = case shown="\"Move FOV\"" w359 {
      selector: w359 -> [w363 _ _ _ _ _ _ _ _ _ _ _ _ _ _ _ _ _ _ _ _ _ _ _ _ _ _ _ _ _]
      tunnel: w358 -> [_ _ _ _ _ _ _ _ _ _ _ _ _ _ _ _ _ _ _ _ _ _ _ _ _ _ _ _ _ _]
      tunnel: w357 -> [_ _ _ _ _ w383 _ _ w419 w431 w459 w478 w484 w499 w547 w556 w565 _ w578 _ _ w604 w612 w632 w653 w679 w697 w718 _ w733]
      tunnel: w356 -> [w362 w366 w368 w373 w378 w386 w409 w411 w421 w437 w460 w479 w496 w501 w548 w558 w567 w569 w571 w593 w597 w600 w614 w636 w656 w680 w699 w714 w729 w735]
      tunnel: [_ _ _ _ _ _ _ _ _ _ _ _ _ _ _ _ _ _ _ _ _ _ _ _ _ _ _ _ _ TRUE] -> w354
      tunnel: [w362 w366 w370 w375 w381 w385 w408 w411 w420 w432 w457 w469 w482 w500 w541 w557 w566 w569 w572 w582 w597 w601 w613 w635 w655 w678 w698 w716 w729 w734] -> w355
      tunnel: w353 -> [w361 w367 w369 w374 w379 w384 w410 w412 w417 w426 w461 w465 w494 w513 w537 w555 w568 w570 w579 w592 w598 w608 w611 w649 w654 w693 w696 w724 w730 w731]
      tunnel: [w361 w367 w369 w374 w379 w384 w410 w412 w416 w427 w456 w467 w494 w513 w537 w551 w568 w570 w576 w592 w598 w603 w611 w634 w654 w677 w696 w724 w730 w731] -> w352
      frame "Typo", Default {
        n232 = Concatenate Strings("Typo: " ("string"), w363) -> (w365:string)
        n233 = One Button Dialog(message=w365) -> ()  [unwired: 1 in, 1 out]
      }
      frame "------Function------" {
      }
      frame "LED On" {
        n234 = call "LED On.vi"("Error In"=w368, "Image Para"=T6 {"Marker"=enum."BF", "Power(Amp)"=55, "set shutter(s)"=0.05, "Cube"=enum."6"}) -> ("Error Out"=w371:errorcluster)  [unwired: 9 in]
        n235 = call "Rendezvous Acquire.vi"("Error In"=w371) -> ("Error Out"=w370:errorcluster)  [unwired: 10 in]
      }
      frame "Rotate U" {
        n236 = call "Rotate U.vi"("Error In"=w373, "Cube"=enum16{"1", "2", "3", "4", "5", "6", "7", "8"}."6") -> ("Error Out"=w376:errorcluster)  [unwired: 9 in]
        n237 = call "Rendezvous Acquire.vi"("Error In"=w376) -> ("Error Out"=w375:errorcluster)  [unwired: 10 in]
      }
      frame "Change Expo" {
        n238 = call "Change Expo.vi"("Error In"=w378, "Expo(s)"=0.05) -> ("Error Out"=w382:errorcluster)  [unwired: 9 in]
        n239 = call "Rendezvous Acquire.vi"("Error In"=w382) -> ("Error Out"=w381:errorcluster)  [unwired: 10 in]
      }
      frame "Rendezvous Wait" {
        n240 = call <vilib>:"Create Rendezvous.vi"("error in (no error)"=w386, "size (2)"=4, "name (unnamed)"="Acquire") -> ("error out"=w395:errorcluster, "rendezvous"=w393:T10)  [unwired: 2 in, 1 out]
        n241 = call <vilib>:"Wait at Rendezvous.vi"("error in (no error)"=w395, "ms timeout (-1)"=10000, "rendezvous"=w393) -> ("error out"=w394:errorcluster, "timed out"=w388:bool, "rendezvous out"=w392:T10)  [unwired: 2 in]
        n242 = call <vilib>:"Destroy Rendezvous.vi"("error in (no error)"=w394, "rendezvous"=w392) -> ("error out"=w387:errorcluster)  [unwired: 4 in, 1 out]
        n243 = case shown="False" w388 {
          tunnel: w387 -> [w397 w401]
          tunnel: [w396 w402] -> w385
          tunnel: w383 -> [_ w400]
          frame False {
            n244 = flat-sequence {
              tunnel: w397 -> [w398]
              tunnel: [w398] -> w396
              frame #0 {
                n245 = Wait (ms)(milliseconds to wait=u32 200) -> ()  [unwired: 1 out]
              }
            }
          }
          frame True {
            n246 = Flush Queue(queue=w400, error in (no error)=w401) -> ()  [unwired: 3 out]
            n247 = xnode "Error Ring"() -> ("error out"=w402:errorcluster)
          }
        }
      }
      frame "LED Off" {
        n248 = call "LED Off.vi"("Error In"=w409) -> ("Error Out"=w408:errorcluster)  [unwired: 10 in]
      }
      frame "------Take Image------" {
      }
      frame "Process Run" {
        n249 = call "Enqueue.vi"("Error In"=w421, "State"="Process Wait", "Queue in"=w419) -> ("Error Out"=w420:errorcluster)  [unwired: 7 in, 1 out]
        n250 = Format Date/Time String(time format string (%c)="%y%m%d_%H%M%S_") -> (date/time string=w414:string)  [unwired: 2 in]
        n251 = Bundle By Name(cluster=w417, "Start Time"=w414, "Take Image Done"=FALSE ("Take Image 8")) -> (w416:T1)
      }
      frame "Process Wait" {
        n252 = call "SEQ Preview Queue.vi"("error in"=w437) -> ("error out"=w434:errorcluster, "SEQ Data"=w436:T5)  [unwired: 9 in]
        n253 = Unbundle By Name(w426) -> ("Current Process"=w425:i32)
        n254 = Unbundle By Name(w436) -> ("Fluidic Process Done?"=w435:bool, "Current Process"=w424:i32)
        n255 = Equal?(x=w425, y=w424) -> (x = y?=w422:bool)
        n256 = Bundle By Name(cluster=w426, "Take Image Done"=w422) -> (w423:T1)
        n257 = Unbundle By Name(w423) -> ("Take Image Done"=w428:bool)
        n258 = Wait (ms)(milliseconds to wait=u32 200) -> ()  [unwired: 1 out]
        n259 = case shown="False" w435 {
          tunnel: w434 -> [w441 w452]
          tunnel: [w441 w452] -> w430
          tunnel: w424 -> [w440 _]
          tunnel: [w439 "Process End"] -> w429
          tunnel: w428 -> [w438 _]
          frame False {
            n260 = case shown="9" w440 {
              tunnel: ["Process Wait" w446 w450] -> w439
              tunnel: w438 -> [_ w443 w447]
              frame Default {
              }
              frame 8 {
                n261 = Select(t="Process Wait", s=w443, f="Take Image") -> (s? t:f=w446:string)
              }
              frame 9 {
                n262 = Select(t="Process Wait", s=w447, f="Take Image") -> (s? t:f=w450:string)
              }
            }
          }
          frame True {
          }
        }
        n263 = Bundle By Name(cluster=w423, "Current Process"=w424) -> (w427:T1)
        n264 = call "Enqueue.vi"("Error In"=w430, "State"=w429, "Queue in"=w431) -> ("Error Out"=w432:errorcluster)  [unwired: 7 in, 1 out]
      }
      frame "Take Image" {
        n265 = call "Enqueue.vi"("Error In"=w460, "State"="Move FOV", "Queue in"=w459) -> ("Error Out"=w457:errorcluster)  [unwired: 7 in, 1 out]
        n266 = Bundle By Name(cluster=w461, "Round Total"=1, "Round Count"=0, "FOV Offset"=i32[] [-500, 500]) -> (w456:T1)
      }
      frame "Move FOV" {
        n267 = Unbundle By Name(w465) -> ("FOV Offset"=w464:i32[], "Round Count"=w463:i32)
        n268 = call "Enqueue.vi"("Error In"=w479, "State"="Move FOV Wait", "Queue in"=w478) -> ("Error Out"=w477:errorcluster)  [unwired: 7 in, 1 out]
        n269 = Index Array(array=w464, index=w463) -> (element=w462:i32)
        n270 = call "SEQ Preview Queue.vi"("error in"=w477) -> ("error out"=w476:errorcluster, "SEQ Data"=w475:T11)  [unwired: 9 in]
        n271 = Unbundle By Name(w475) -> ("Flower Position"=w474:i32[])
        n272 = Index Array(array=w474) -> (element=w473:i32)  [unwired: 1 in]
        n273 = Add(x=w473, y=w462) -> (x+y=w472:i32)
        n274 = Number To Decimal String(number=w472) -> (decimal integer string=w471:string)  [unwired: 1 in]
        n275 = Tick Count (ms)() -> (millisecond timer value=w466:u32)
        n276 = call "Move Axis 1.vi"("Error In"=w476, "Position"=w471) -> ("Error Out"=w470:errorcluster)  [unwired: 9 in]
        n277 = Bundle By Name(cluster=w465, "Tick Count"=w466) -> (w467:T1)
        n278 = flat-sequence {
          tunnel: w470 -> [w480]
          tunnel: [w480] -> w469
          frame #0 {
            n279 = Wait (ms)(milliseconds to wait=u32 1000) -> ()  [unwired: 1 out]
          }
        }
      }
      frame "Move FOV Wait" {
        n280 = Unbundle By Name(w494) -> ("Tick Count"=w493:u32)
        n281 = call "SEQ Preview Queue.vi"("error in"=w496) -> ("error out"=w486:errorcluster, "SEQ Data"=w495:T12)  [unwired: 9 in]
        n282 = Tick Count (ms)() -> (millisecond timer value=w492:u32)
        n283 = Unbundle By Name(w495) -> ("Arrived?"=w488:bool)
        n284 = Subtract(x=w492, y=w493) -> (x-y=w491:u32)
        n285 = Greater?(x=w491, y=u32 60000) -> (0:w489:bool)
        n286 = Or(x=w489, y=w488) -> (x .or. y?=w487:bool)
        n287 = case shown="True" w487 {
          tunnel: ["Move FOV Wait" "Snap"] -> w483
          frame False {
          }
          frame True {
          }
        }
        n288 = Wait (ms)(milliseconds to wait=u32 100) -> ()  [unwired: 1 out]
        n289 = call "Enqueue.vi"("Error In"=w486, "State"=w483, "Queue in"=w484) -> ("Error Out"=w482:errorcluster)  [unwired: 7 in, 1 out]
      }
      frame "Snap" {
        n290 = call "Snap.vi"("Error In"=w501) -> ("Error Out"=w512:errorcluster)  [unwired: 10 in]
        n291 = call "Rendezvous Snap.vi"("Error In"=w512) -> ("Error Out"=w511:errorcluster)  [unwired: 10 in]
        n292 = call <vilib>:"Create Rendezvous.vi"("error in (no error)"=w511, "size (2)"=2, "name (unnamed)"="Snap") -> ("error out"=w510:errorcluster, "rendezvous"=w508:T10)  [unwired: 2 in, 1 out]
        n293 = call <vilib>:"Wait at Rendezvous.vi"("error in (no error)"=w510, "ms timeout (-1)"=5000, "rendezvous"=w508) -> ("error out"=w509:errorcluster, "timed out"=w502:bool, "rendezvous out"=w507:T10)  [unwired: 2 in]
        n294 = call <vilib>:"Destroy Rendezvous.vi"("error in (no error)"=w509, "rendezvous"=w507) -> ("error out"=w503:errorcluster)  [unwired: 4 in, 1 out]
        n295 = case shown="False" w502 {
          tunnel: w503 -> [w517 _]
          tunnel: [w516 w518] -> w500
          tunnel: w499 -> [w515 _]
          frame False {
            n296 = call "Enqueue.vi"("Error In"=w517, "State"="Save Image", "Queue in"=w515) -> ("Error Out"=w516:errorcluster)  [unwired: 7 in, 1 out]
          }
          frame True {
            n297 = xnode "Error Ring"() -> ("error out"=w518:errorcluster)
          }
        }
      }
      frame "Save Image" {
        n298 = call "Enqueue.vi"("Error In"=w548, "State"="Next", "Queue in"=w547) -> ("Error Out"=w531:errorcluster)  [unwired: 7 in, 1 out]
        n299 = call "SEQ Preview Queue.vi"("error in"=w531) -> ("error out"=w530:errorcluster, "SEQ Data"=w529:T13)  [unwired: 9 in]
        n300 = Unbundle By Name(w529) -> ("Folder Path"=w528:path)
        n301 = Unbundle By Name(w537) -> ("Start Time"=w526:string, "Current Process"=w525:i32, "Round Count"=w527:i32)
        n302 = Build Path(base path=w528, name or relative path="Flow Field") -> (appended path=w539:path)
        n303 = call "Create Folder.vi"("error in"=w530, "Path in"=w539) -> ("error out"=w540:errorcluster, "Path out"=w538:path)  [unwired: 8 in]
        n304 = Number To Decimal String(number=w527) -> (decimal integer string=w532:string)  [unwired: 1 in]
        n305 = Number To Decimal String(number=w525) -> (decimal integer string=w524:string)  [unwired: 1 in]
        n306 = Concatenate Strings(w526, w524, "_FOV", w532, ".tif" ("string")) -> (w536:string)
        n307 = Build Path(base path=w538, name or relative path=w536) -> (appended path=w535:path)
        n308 = call "SEQ Preview Queue.vi"("error in"=w540) -> ("error out"=w544:errorcluster, "SEQ Data"=w545:T14)  [unwired: 9 in]
        n309 = Unbundle By Name(w545) -> ("Image Ref"=w543:T15)
        n310 = call-poly "IMAQ Write File 2"("error in (no error)"=w544, "File Path"=w535, "Image"=w543) -> ("error out"=w541:errorcluster)  [unwired: 7 in, 1 out]
      }
      frame "Next" {
        n311 = Unbundle By Name(w555) -> ("Round Total"=w554:i32, "Round Count"=w552:i32)
        n312 = Equal?(x=w554, y=w552) -> (x = y?=w553:bool)
        n313 = case shown="True" w553 {
          tunnel: ["Move FOV" "Process Wait"] -> w549
          tunnel: w552 -> [w560 _]
          tunnel: [w559 0] -> w550
          frame False {
            n314 = Increment(x=w560) -> (x+1=w559:i32)
          }
          frame True {
          }
        }
        n315 = Bundle By Name(cluster=w555, "Round Count"=w550) -> (w551:T1)
        n316 = call "Enqueue.vi"("Error In"=w558, "State"=w549, "Queue in"=w556) -> ("Error Out"=w557:errorcluster)  [unwired: 7 in, 1 out]
      }
      frame "Process End" {
        n317 = call "Enqueue.vi"("Error In"=w567, "State"="LED Off", "Queue in"=w565) -> ("Error Out"=w566:errorcluster)  [unwired: 7 in, 1 out]
      }
      frame "------Home------" {
      }
      frame "Home" {
        n318 = call "Enqueue.vi"("Error In"=w571, "State"="Home Wait", "Queue in"=w578) -> ("Error Out"=w574:errorcluster)  [unwired: 7 in, 1 out]
        n319 = call "Home.vi"("Error In"=w574) -> ("Error Out"=w573:errorcluster)  [unwired: 10 in]
        n320 = flat-sequence {
          tunnel: w573 -> [w580]
          tunnel: [w580] -> w572
          frame #0 {
            n321 = Wait (ms)(milliseconds to wait=u32 1000) -> ()  [unwired: 1 out]
          }
        }
        n322 = Tick Count (ms)() -> (millisecond timer value=w575:u32)
        n323 = Bundle By Name(cluster=w579, "Tick Count"=w575) -> (w576:T1)
      }
      frame "Home Wait" {
        n324 = call "SEQ Preview Queue.vi"("error in"=w593) -> ("error out"=w584:errorcluster, "SEQ Data"=w587:T12)  [unwired: 9 in]
        n325 = Unbundle By Name(w592) -> ("Tick Count"=w590:u32)
        n326 = Tick Count (ms)() -> (millisecond timer value=w591:u32)
        n327 = Unbundle By Name(w587) -> ("Arrived?"=w585:bool)
        n328 = Subtract(x=w591, y=w590) -> (x-y=w589:u32)
        n329 = Greater Or Equal?(x=w589, y=u32 180000) -> (x >= y?=w586:bool)
        n330 = Or(x=w586, y=w585) -> (x .or. y?=w583:bool)
        n331 = case shown="True" w583 {
          tunnel: w584 -> [w594 w596]
          tunnel: [w594 w595] -> w582
          frame False {
          }
          frame True {
            n332 = call "Display Message to User3"("error in (no error)"=w596) -> ("error out"=w595:errorcluster)  [unwired: 9 in, 1 out]
          }
        }
      }
      frame "------Locate------" {
      }
      frame "Go Reference" {
        n333 = call "Busy.vi"("Error In"=w600) -> ("Error Out"=w599:errorcluster)  [unwired: 10 in]
        n334 = call "Enqueue.vi"("Error In"=w599, "State"="Go Reference Wait", "Queue in"=w604) -> ("Error Out"=w606:errorcluster)  [unwired: 7 in, 1 out]
        n335 = call "Go Reference.vi"("Error In"=w606) -> ("Error Out"=w605:errorcluster)  [unwired: 10 in]
        n336 = flat-sequence {
          tunnel: w605 -> [w609]
          tunnel: [w609] -> w601
          frame #0 {
            n337 = Wait (ms)(milliseconds to wait=u32 1000) -> ()  [unwired: 1 out]
          }
        }
        n338 = Tick Count (ms)() -> (millisecond timer value=w602:u32)
        n339 = Bundle By Name(cluster=w608, "Tick Count"=w602) -> (w603:T1)
      }
      frame "Go Reference Wait" {
        n340 = call "SEQ Preview Queue.vi"("error in"=w614) -> ("error out"=w616:errorcluster, "SEQ Data"=w617:T12)  [unwired: 9 in]
        n341 = Tick Count (ms)() -> (millisecond timer value=w624:u32)
        n342 = Unbundle By Name(w611) -> ("Tick Count"=w623:u32)
        n343 = Unbundle By Name(w617) -> ("Arrived?"=w615:bool)
        n344 = Subtract(x=w624, y=w623) -> (x-y=w622:u32)
        n345 = Greater Or Equal?(x=w622, y=u32 60000) -> (x >= y?=w620:bool)
        n346 = Wait (ms)(milliseconds to wait=u32 100) -> ()  [unwired: 1 out]
        n347 = Or(x=w620, y=w615) -> (x .or. y?=w619:bool)
        n348 = case shown="True" w619 {
          tunnel: ["Go Reference Wait" "Locating Triangle"] -> w618
          frame False {
          }
          frame True {
          }
        }
        n349 = call "Enqueue.vi"("Error In"=w616, "State"=w618, "Queue in"=w612) -> ("Error Out"=w613:errorcluster)  [unwired: 7 in, 1 out]
      }
      frame "Locating Triangle" {
        n350 = call "Enqueue.vi"("Error In"=w636, "State"="Locating Triangle Wait", "Queue in"=w632) -> ("Error Out"=w631:errorcluster)  [unwired: 7 in, 1 out]
        n351 = call "SEQ Preview Queue.vi"("error in"=w631) -> ("error out"=w628:errorcluster, "SEQ Data"=w630:T13)  [unwired: 9 in]
        n352 = Unbundle By Name(w630) -> ("Folder Path"=w629:path)
        n353 = Build Path(base path=w629, name or relative path="Locating Chip") -> (appended path=w642:path)
        n354 = call "Create Folder.vi"("error in"=w628, "Path in"=w642) -> ("error out"=w640:errorcluster, "Path out"=w641:path)  [unwired: 8 in]
        n355 = Bundle By Name(cluster=T9 {"Image Path"=path "", "Start Offset"=0, "Template Path"=path "", "Disable Fine Search"=FALSE, "ROI"={"Global Rectangle"=[], "Contours"=[]}} ("Match Data"), "Template Path"=path "C:/MiCareo/MiSelectMiControl/PARAMETER/IMAGE/20180613.png" ("File Path"), "Start Offset"=0, "Disable Fine Search"=TRUE, "Image Path"=w641, "ROI"=T8 {"Global Rectangle"=[0, 0, 2560, 2160], "Contours"=[{"ID"=enum."External", "Type"=3, "Coordinates"=[0, 0, 2560, 2160, 0]}]}) -> (w637:T9)
        n356 = Tick Count (ms)() -> (millisecond timer value=w633:u32)
        n357 = Bundle By Name(cluster=w649, "Tick Count"=w633) -> (w634:T1)
        n358 = call "Match Pattern.vi"("Error In"=w640, "Match Data"=w637) -> ("Error Out"=w645:errorcluster)  [unwired: 9 in]
        n359 = flat-sequence {
          tunnel: w645 -> [w651]
          tunnel: [w651] -> w635
          frame #0 {
            n360 = Wait (ms)(milliseconds to wait=u32 1000) -> ()  [unwired: 1 out]
          }
        }
      }
      frame "Locating Triangle Wait" {
        n361 = call "SEQ Preview Queue.vi"("error in"=w656) -> ("error out"=w658:errorcluster, "SEQ Data"=w659:T11)  [unwired: 9 in]
        n362 = Tick Count (ms)() -> (millisecond timer value=w665:u32)
        n363 = Unbundle By Name(w654) -> ("Tick Count"=w664:u32)
        n364 = Unbundle By Name(w659) -> ("Match Done?"=w657:bool)
        n365 = Subtract(x=w665, y=w664) -> (x-y=w663:u32)
        n366 = Greater Or Equal?(x=w663, y=u32 180000) -> (x >= y?=w652:bool)
        n367 = Or(x=w652, y=w657) -> (x .or. y?=w661:bool)
        n368 = Wait (ms)(milliseconds to wait=u32 100) -> ()  [unwired: 1 out]
        n369 = case shown="True" w661 {
          tunnel: ["Locating Triangle Wait" w669] -> w660
          tunnel: w652 -> [_ w668]
          frame False {
          }
          frame True {
            n370 = case shown="True" w668 {
              tunnel: ["Locating Flower" "Locating End"] -> w669
              frame False {
              }
              frame True {
              }
            }
          }
        }
        n371 = call "Enqueue.vi"("Error In"=w658, "State"=w660, "Queue in"=w653) -> ("Error Out"=w655:errorcluster)  [unwired: 7 in, 1 out]
      }
      frame "Locating Flower" {
        n372 = call "Enqueue.vi"("Error In"=w680, "State"="Locating Flower Wait", "Queue in"=w679) -> ("Error Out"=w675:errorcluster)  [unwired: 7 in, 1 out]
        n373 = call "SEQ Preview Queue.vi"("error in"=w675) -> ("error out"=w672:errorcluster, "SEQ Data"=w674:T13)  [unwired: 9 in]
        n374 = Unbundle By Name(w674) -> ("Folder Path"=w673:path)
        n375 = Build Path(base path=w673, name or relative path="Locating Chip") -> (appended path=w685:path)
        n376 = call "Create Folder.vi"("error in"=w672, "Path in"=w685) -> ("error out"=w686:errorcluster, "Path out"=w684:path)  [unwired: 8 in]
        n377 = Bundle By Name(cluster=T9 {"Image Path"=path "", "Start Offset"=0, "Template Path"=path "", "Disable Fine Search"=FALSE, "ROI"={"Global Rectangle"=[], "Contours"=[]}} ("Match Data"), "Template Path"=path "C:/MiCareo/MiSelectMiControl/PARAMETER/IMAGE/Chip/Chip20160427.png" ("File Path"), "Start Offset"=0, "Disable Fine Search"=FALSE, "Image Path"=w684, "ROI"=T8 {"Global Rectangle"=[1030, 830, 1530, 1330], "Contours"=[{"ID"=enum."External", "Type"=3, "Coordinates"=[1030, 830, 1530, 1330, 0]}]}) -> (w681:T9)
        n378 = Tick Count (ms)() -> (millisecond timer value=w676:u32)
        n379 = Bundle By Name(cluster=w693, "Tick Count"=w676) -> (w677:T1)
        n380 = call "Match Pattern.vi"("Error In"=w686, "Match Data"=w681) -> ("Error Out"=w690:errorcluster)  [unwired: 9 in]
        n381 = flat-sequence {
          tunnel: w690 -> [w695]
          tunnel: [w695] -> w678
          frame #0 {
            n382 = Wait (ms)(milliseconds to wait=u32 1000) -> ()  [unwired: 1 out]
          }
        }
      }
      frame "Locating Flower Wait" {
        n383 = call "SEQ Preview Queue.vi"("error in"=w699) -> ("error out"=w701:errorcluster, "SEQ Data"=w702:T11)  [unwired: 9 in]
        n384 = Unbundle By Name(w696) -> ("Tick Count"=w708:u32)
        n385 = Unbundle By Name(w702) -> ("Match Done?"=w700:bool)
        n386 = Tick Count (ms)() -> (millisecond timer value=w709:u32)
        n387 = Subtract(x=w709, y=w708) -> (x-y=w707:u32)
        n388 = Greater Or Equal?(x=w707, y=u32 180000) -> (x >= y?=w705:bool)
        n389 = Or(x=w705, y=w700) -> (x .or. y?=w704:bool)
        n390 = case shown="True" w704 {
          tunnel: ["Locating Flower Wait" "Locating End"] -> w703
          frame False {
          }
          frame True {
          }
        }
        n391 = Wait (ms)(milliseconds to wait=u32 100) -> ()  [unwired: 1 out]
        n392 = call "Enqueue.vi"("Error In"=w701, "State"=w703, "Queue in"=w697) -> ("Error Out"=w698:errorcluster)  [unwired: 7 in, 1 out]
      }
      frame "Locating End" {
        n393 = call "Unbusy.vi"("Error In"=w714) -> ("Error Out"=w713:errorcluster)  [unwired: 10 in]
        n394 = call "Enqueue.vi"("Error In"=w713, "State"="LED Off", "Queue in"=w718) -> ("Error Out"=w719:errorcluster)  [unwired: 7 in, 1 out]
        n395 = call "SEQ Preview Queue.vi"("error in"=w719) -> ("error out"=w717:errorcluster, "SEQ Data"=w722:T11)  [unwired: 9 in]
        n396 = Unbundle By Name(w722) -> ("Match Score"=w721:dbl)
        n397 = Greater?(x=w721, y=300.0) -> (0:w715:bool)
        n398 = case shown="False" w715 {
          tunnel: w717 -> [w726 w728]
          tunnel: [w725 w727] -> w716
          frame False {
            n399 = call "Display Message to User"("error in (no error)"=w726) -> ("error out"=w725:errorcluster)  [unwired: 9 in, 1 out]
          }
          frame True {
            n400 = call "Display Message to User2"("error in (no error)"=w728) -> ("error out"=w727:errorcluster)  [unwired: 9 in, 1 out]
          }
        }
      }
      frame "------Close------" {
      }
      frame "Close" {
        n401 = Release Queue(queue=w733, error in (no error)=w735) -> (error out=w734:errorcluster)  [unwired: 1 in, 2 out]
      }
    }
  }
  n402 = Merge Errors(w21, w20, w7) -> (w18:errorcluster)
  n403 = Unregister For Events(event registration refnum=w19, error in=w18) -> (error out=w17:errorcluster)
  n404 = Destroy User Event(user event=w12, error in=w17) -> (error out=→"error out":errorcluster)
